vi "Pass Dictionary Argument.vi"() -> ()   [LabVIEW 2019, in "OPI.lvclass"]
uses:
  OPI.lvclass
  Typedefs/Cmd Line Mode.ctl
  To Pythonic/To Pythonic - String.vi
  To Pythonic/To Pythonic - Integer.vi
  To Pythonic/To Pythonic - Float.vi
  To Pythonic/To Pythonic - Dictionary.vi
  Get Return/Get Return - Pythonic.vi
panel:
  out "Output Dictionary":string
  out "Input Dictionary":string
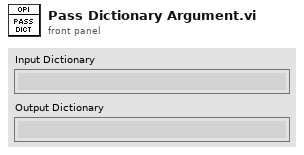
[diagram p1: front panel]
types:
  T1 = typedef "OPI.lvclass/Cmd Line Mode.ctl" = enum16{"Debug", "Hidden"}
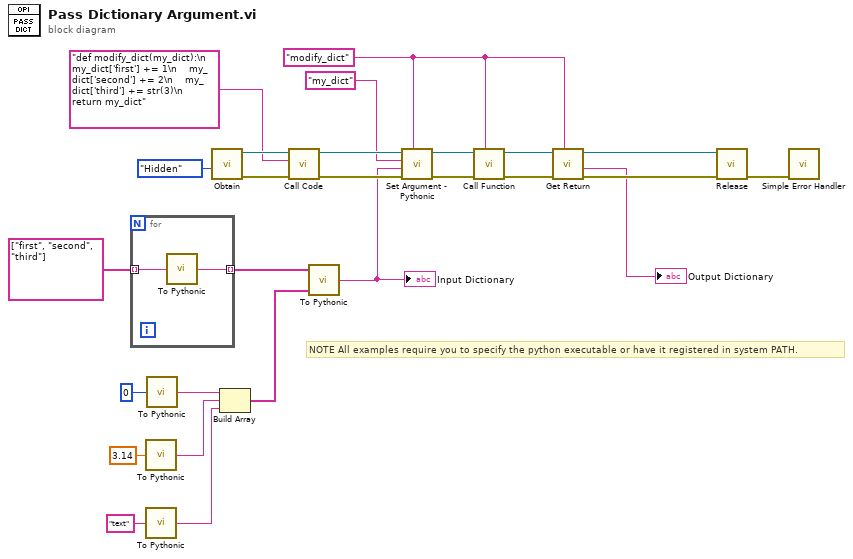
[diagram p0: block diagram]
diagram:
  w2 = "modify_dict" ("Function Name")
  # "NOTE All examples require you to specify the python executable or have it registered in system PATH."
  n1 = for {
    tunnel: string[] ["first", "second", "third"] ("String") -> [w28] mode=indexing
    tunnel: [w27] -> w11 mode=indexing
    n2 = call-poly "To Pythonic.vi"("String"=w28) -> ("Pythonic Value"=w27:string)  [unwired: 4 in]
  }
  n3 = call-poly "To Pythonic.vi"("Float"=3.14) -> ("Pythonic Value"=w6:string)  [unwired: 4 in]
  n4 = call-poly "To Pythonic.vi"("String"="text") -> ("Pythonic Value"=w5:string)  [unwired: 4 in]
  n5 = call-poly "To Pythonic.vi"("Integer"=i64 0) -> ("Pythonic Value"=w7:string)  [unwired: 4 in]
  n6 = call "Obtain.vi"("Cmd Line Mode (Hidden)"=Cmd_Line_Mode."Hidden") -> ("Error Out"=w25:errorcluster, "OPI Ref"=w26:refnum<data-value>)  [unwired: 9 in]
  n7 = Build Array(w7, w6, w5) -> (w4:string[])
  n8 = call "Call Code.vi"("Error In"=w25, "Pythonic Code"="def modify_dict(my_dict):\n    my_dict['first'] += 1\n    my_dict['second'] += 2\n    my_dict['third'] += str(3)\n    return my_dict", "OPI Ref"=w26) -> ("Error Out"=w15:errorcluster, "OPI Ref"=w18:refnum<data-value>)  [unwired: 7 in]
  n9 = call-poly "To Pythonic.vi"("Pythonic Values"=w4, "Pythonic Keys"=w11) -> ("Dictionary"=w14:string)  [unwired: 3 in]
  "Input Dictionary" <- w14
  n10 = call "Set Argument - Pythonic.vi"("Function Name"=w2, "Error In"=w15, "Pythonic Value"=w14, "Argument"="my_dict", "OPI Ref"=w18) -> ("Error Out"=w16:errorcluster, "OPI Ref"=w17:refnum<data-value>)  [unwired: 5 in]
  n11 = call "Call Function.vi"("Function Name"=w2, "Error In"=w16, "OPI Ref"=w17) -> ("Error Out"=w21:errorcluster, "OPI Ref"=w22:refnum<data-value>)  [unwired: 7 in]
  n12 = call-poly "Get Return.vi"("Function Name"=w2, "Error In"=w21, "OPI Ref"=w22) -> ("Error Out"=w20:errorcluster, "Pythonic Return Value"=→"Output Dictionary":string, "OPI Ref"=w24:refnum<data-value>)  [unwired: 6 in]
  n13 = call "Release.vi"("Error In"=w20, "OPI Ref"=w24) -> ("Error Out"=w19:errorcluster)  [unwired: 9 in]
  n14 = call <vilib>:"Simple Error Handler.vi"("error in (no error)"=w19) -> ()  [unwired: 4 in, 5 out]
